vi "UHR-Fleezers Control (host) - 11.9b.vi"() -> ()   [LabVIEW 2014] (continued)
        n1088 = xnode "Read/Write Control"("FPGA VI Reference In"=w1466, "error in"=w1467, "+ phase (APD 1 Gate)"=w1464) -> ("error out"=w1465:errorcluster)  [unwired: 1 out]
      }
      event "+ phase (APD 2 Gate)", "- phase (APD 2 Gate)": Value Change {
        n1089 = event-data() -> ()  [unwired: 7 out]
        n1090 = local read "Phase Adj. (APD 2 Gate)"() -> (w1472:i16)
        n1091 = Negate(x=w1472) -> (-x=w1480:i16)
        n1092 = Select(t=w1480, s="- phase (APD 2 Gate)", f=w1472) -> (s? t:f=w1479:i16)
        n1093 = Or(x="- phase (APD 2 Gate)", y="+ phase (APD 2 Gate)") -> (x .or. y?=w1475:bool)
        n1094 = xnode "Read/Write Control"("FPGA VI Reference In"=w1482, "error in"=w1481, "Phase count adjustment (APD 2 Gate)"=w1479) -> ("FPGA VI Reference Out"=w1477:T19, "error out"=w1478:errorcluster)
        n1095 = xnode "Read/Write Control"("FPGA VI Reference In"=w1477, "error in"=w1478, "+ phase (APD 2 Gate)"=w1475) -> ("error out"=w1476:errorcluster)  [unwired: 1 out]
      }
      event "Phase Adj. (APD Acq)", "+ phase (APD Acq)", "- phase (APD Acq)": Value Change {
        n1096 = event-data() -> ()  [unwired: 7 out]
        n1097 = local read "Phase Adj. (APD Acq)"() -> (w1485:i16)
        n1098 = Negate(x=w1485) -> (-x=w1491:i16)
        n1099 = Select(t=w1491, s="+ phase (APD Acq)", f=w1485) -> (s? t:f=w1490:i16)
        n1100 = Or(x="+ phase (APD Acq)", y="- phase (APD Acq)") -> (x .or. y?=w1486:bool)
        n1101 = xnode "Read/Write Control"("FPGA VI Reference In"=w1493, "error in"=w1492, "Phase Count Adjustment (APD Acq)"=w1490) -> ("FPGA VI Reference Out"=w1488:T19, "error out"=w1489:errorcluster)
        n1102 = xnode "Read/Write Control"("FPGA VI Reference In"=w1488, "error in"=w1489, "+ phase (APD Acq)"=w1486) -> ("error out"=w1487:errorcluster)  [unwired: 1 out]
      }
      event "Phase adj. (GI)", "+ phase (GI)", "- phase (GI)": Value Change {
        n1103 = event-data() -> ()  [unwired: 7 out]
        n1104 = Negate(x="Phase adj. (GI)") -> (-x=w1502:i16)
        n1105 = Select(t=w1502, s="+ phase (GI)", f="Phase adj. (GI)") -> (s? t:f=w1501:i16)
        n1106 = Or(x="+ phase (GI)", y="- phase (GI)") -> (x .or. y?=w1497:bool)
        n1107 = xnode "Read/Write Control"("FPGA VI Reference In"=w1504, "error in"=w1503, "Phase count adjustment (GI)"=w1501) -> ("FPGA VI Reference Out"=w1499:T19, "error out"=w1500:errorcluster)
        n1108 = xnode "Read/Write Control"("FPGA VI Reference In"=w1499, "error in"=w1500, "+ phase (GI)"=w1497) -> ("error out"=w1498:errorcluster)  [unwired: 1 out]
      }
      event "Phase adj. (GI) 2", "+ phase (GI) 2", "- phase (GI) 2": Value Change {
        n1109 = event-data() -> ()  [unwired: 7 out]
        n1110 = Negate(x="Phase adj. (GI) 2") -> (-x=w1513:i16)
        n1111 = Select(t=w1513, s="+ phase (GI) 2", f="Phase adj. (GI) 2") -> (s? t:f=w1512:i16)
        n1112 = Or(x="+ phase (GI) 2", y="- phase (GI) 2") -> (x .or. y?=w1508:bool)
        n1113 = xnode "Read/Write Control"("FPGA VI Reference In"=w1515, "error in"=w1514, "Phase count adjustment (GI) 2"=w1512) -> ("FPGA VI Reference Out"=w1510:T19, "error out"=w1511:errorcluster)
        n1114 = xnode "Read/Write Control"("FPGA VI Reference In"=w1510, "error in"=w1511, "+ phase (GI) 2"=w1508) -> ("error out"=w1509:errorcluster)  [unwired: 1 out]
      }
      event "Phase adj. (Green FB)", "- phase (Green FB)", "+ phase (Green FB)": Value Change {
        n1115 = event-data() -> ()  [unwired: 7 out]
        n1116 = Negate(x="Phase adj. (Green FB)") -> (-x=w1524:i16)
        n1117 = Select(t=w1524, s="+ phase (Green FB)", f="Phase adj. (Green FB)") -> (s? t:f=w1523:i16)
        n1118 = Or(x="+ phase (Green FB)", y="- phase (Green FB)") -> (x .or. y?=w1519:bool)
        n1119 = xnode "Read/Write Control"("FPGA VI Reference In"=w1526, "error in"=w1525, "Phase count adjustment (Green FB)"=w1523) -> ("FPGA VI Reference Out"=w1521:T19, "error out"=w1522:errorcluster)
        n1120 = xnode "Read/Write Control"("FPGA VI Reference In"=w1521, "error in"=w1522, "+ phase (Green FB)"=w1519) -> ("error out"=w1520:errorcluster)  [unwired: 1 out]
      }
      event "Invert APD Gate", "APD Gate ON Count", "APD Gate OFF Count", "APD Gate", "APD Integration Time (s)", "APD 1 AO Mult.", "APD 2 AO Mult.", "On one out of X cycles": Value Change {
        n1121 = event-data() -> ()  [unwired: 7 out]
        n1122 = Add(x="GI Frequency, ON count", y="GI Frequency, OFF count") -> (x+y=w1530:u32)
        n1123 = Add(x="APD Gate ON Count", y="APD Gate OFF Count") -> (x+y=w1543:u32)
        n1124 = Multiply(x="On one out of X cycles", y=w1530) -> (x*y=w1527:u32)
        "Green FB Count" <- w1527
        n1125 = Subtract(x=w1527, y="GI Frequency, ON count") -> (x-y=w1528:u32)
        n1126 = Multiply(x=w1543, y="On one out of X cycles") -> (x*y=w1542:u32)
        n1127 = Subtract(x=w1542, y="APD Gate ON Count") -> (x-y=w1541:u32)
        n1128 = local read "DMA Update Period (s)"() -> (w1544:dbl)
        n1129 = Multiply(x="APD Integration Time (s)", y=40000000.0) -> (x*y=w1549:dbl)
        n1130 = Reciprocal(x="APD Integration Time (s)") -> (1/x=→"APD Acq Rate (Hz)":dbl)
        n1131 = To Unsigned Long Integer(number=w1549) -> (unsigned 32bit integer=w1533:u32)
        "APD Int. Count" <- w1533
        n1132 = xnode "Read/Write Control"("FPGA VI Reference In"=w1553, "error in"=w1552, "Invert APD Gate"="Invert APD Gate", "APD Gate ON Count"="APD Gate ON Count", "APD Gate OFF Count"=w1541, "APD Acq Rate Count"=w1533, "APD Gate Operating Mode"="APD Gate", "APD 1 AO scale factor"="APD 1 AO Mult.", "APD 2 AO scale factor"="APD 2 AO Mult.", "Green interlace ON count"="GI Frequency, ON count", "Green interlace OFF count"=w1528, "Green interlace ON count 2"="GI Frequency, ON count", "Green interlace OFF count 2"=w1528, "Green FB Count"=w1527) -> ("error out"=w1551:errorcluster)  [unwired: 1 out]
        n1133 = Divide(x=w1544, y="APD Integration Time (s)") -> (x/y=w1547:dbl)
        n1134 = Multiply(x=2.0, y=w1547) -> (x*y=w1546:dbl)
        n1135 = local write "APD Samples/FIFO Acq."(w1547) -> ()
        n1136 = local write "APD Elements/DMA read"(w1546) -> ()
      }
      event "Number of F/B Scans (AOD)", "Scan Speed (nm/s)", "Scan BD", "Initial D (MHz)", "Step Size (nm)", "Scan Range (nm)", "Wiggle amp 1 (units?)": Value Change {
        w1615 = 123.0  # AOM cal (nm/MHz)
        n1137 = event-data() -> ()  [unwired: 7 out]
        n1138 = local read "BD 1 Frequency 1 (MHz)"() -> (w1598:dbl)
        n1139 = local read "AOM X Cal (nm/MHz)"() -> (w1590:dbl)
        n1140 = local read "BD 2 Frequency 1 (MHz)"() -> (w1604:dbl)
        n1141 = local read "X RF Frequency Limits (MHz)"() -> (w1602:T16)
        n1142 = local read "Y RF Frequency Limits (MHz)"() -> (w1599:T16)
        n1143 = Negate(x="Scan Range (nm)") -> (-x=w1568:dbl)
        n1144 = Divide(x=w1568, y=w1590) -> (x/y=w1572:dbl)
        n1145 = Select(t=w1602, s="Scan BD", f=w1599) -> (s? t:f=w1601:T16)
        n1146 = Select(t=w1598, s="Scan BD", f=w1604) -> (s? t:f=w1603:dbl)
        n1147 = Unbundle By Name(w1601) -> ("Maximum"=w1610:dbl, "Minimum"=w1609:dbl)
        n1148 = Add(x=w1572, y=w1603) -> (x+y=w1607:dbl)
        n1149 = Divide(x=w1568, y="Step Size (nm)") -> (x/y=w1587:dbl)
        n1150 = Divide(x="Step Size (nm)", y=w1590) -> (x/y=w1596:dbl)
        n1151 = Absolute Value(x=w1587) -> (abs(x)=w1571:dbl)
        n1152 = Sign(1:w1568) -> (0:w1569:dbl)
        n1153 = In Range and Coerce(upper limit=w1610, x=w1607, lower limit=w1609) -> (coerced(x)=w1606:dbl, In Range?=w1608:bool)
        n1154 = To Unsigned Quad Integer(1:w1571) -> (0:w1586:u64)
        "Scan steps (AOD)" <- w1586
        n1155 = call "IR AOM freq to word.vi"("Frequency In (MHz)"=w1596) -> ("Frequency Word Out (double)"=w1593:dbl)
        n1156 = Multiply(x=w1569, y=w1593) -> (x*y=w1570:dbl)
        n1157 = Subtract(x=w1607, y=w1606) -> (x-y=w1605:dbl)
        n1158 = To Quad Integer(1:w1570) -> (0:w1592:i64)
        "Incr. int (AOD)" <- w1592
        n1159 = Subtract(x=w1572, y=w1605) -> (x-y=w1591:dbl)
        "Scan Range (MHz)" <- w1591
        n1160 = Select(t=w1572, s=w1608, f=w1591) -> (s? t:f=w1611:dbl)
        n1161 = Multiply(x=w1591, y=w1590) -> (x*y=w1589:dbl)
        n1162 = Decrement(x=w1586) -> (x-1=w1639:u64)
        n1163 = Negate(x=w1589) -> (-x=w1585:dbl)
        n1164 = local write "Scan Range (nm)"(w1585) -> ()
        n1165 = Divide(x=w1611, y=w1639) -> (x/y=w1595:dbl)
        "Scan Increment (MHz)" <- w1595
        n1166 = call "IR AOM freq to word.vi"("Frequency In (MHz)"=w1595) -> ("Frequency Word Out (double)"=w1594:dbl)
        n1167 = Divide(x="Step Size (nm)", y="Scan Speed (nm/s)") -> (x/y=w1582:dbl)
        n1168 = To Quad Integer(1:w1594) -> ()  [unwired: 1 out]
        n1169 = local read "Number Interlace Sets"() -> (w1566:u8)
        n1170 = local read "AI Count (ticks)"() -> (w1567:u32)
        n1171 = local read "Total Counts (ticks)"() -> (w1565:u32)
        n1172 = local read "# Samples/trap"() -> (w1597:u32)
        n1173 = Multiply(x=w1567, y=w1566) -> (x*y=w1564:u32)
        n1174 = Divide(x=w1565, y=w1564) -> (x/y=w1563:dbl)
        n1175 = Select(t=w1598, s="Scan BD", f=w1604) -> (s? t:f=w1636:dbl)
        "Initial freq. (MHz)" <- w1636
        n1176 = Add(x=w1611, y=w1636) -> (x+y=→"Final freq. (MHz)":dbl)
        n1177 = Divide(x=w1565, y=40000000.0) -> (x/y=w1581:dbl)
        n1178 = Divide(x=w1582, y=w1581) -> (x/y=w1580:dbl)
        n1179 = To Unsigned Quad Integer(1:w1580) -> (0:w1555:u64)
        n1180 = Quotient & Remainder(x=w1555, y=u64 2) -> (x-y*floor(x/y)=w1559:u64)  [unwired: 1 out]
        n1181 = Equal?(x=w1559, y=u64 0) -> (x = y?=w1557:bool)
        n1182 = Decrement(x=w1555) -> (x-1=w1556:u64)
        n1183 = Select(t=w1555, s=w1557, f=w1556) -> (s? t:f=w1554:u64)
        "Cycles/step (AOD)" <- w1554
        n1184 = xnode "Read/Write Control"("FPGA VI Reference In"=w1647, "error in"=w1646, "Scan steps"=w1586, "Number of scans"="Number of F/B Scans (AOD)", "Cycles per step"=w1554, "Scan freq.  increment"=w1592, "Scan BD"="Scan BD") -> ("error out"=w1645:errorcluster)  [unwired: 1 out]
        n1185 = Multiply(x=w1586, y=w1554) -> (x*y=w1640:u64)
        n1186 = Multiply(x=w1640, y=u64 2) -> (x*y=w1562:u64)
        n1187 = Multiply(x=w1563, y=w1562) -> (x*y=w1561:dbl)
        "Data points/scan (f/b)" <- w1561
        n1188 = Multiply(x=w1561, y="Number of F/B Scans (AOD)") -> (x*y=w1643:dbl)
        "Data points/scans" <- w1643
        n1189 = Divide(x=w1643, y=w1597) -> (x/y=→"N sets should be saved":dbl)
        n1190 = Multiply(x=w1640, y=w1581) -> (x*y=w1579:dbl)
        "Time/Scan (s) (AOD)" <- w1579
        n1191 = Select(t=w1611, s="Scan BD", f=0.0) -> (s? t:f=w1637:dbl)
        n1192 = Select(t=0.0, s="Scan BD", f=w1611) -> (s? t:f=w1633:dbl)
        n1193 = local read "BD 2 Frequency 2 (MHz)"() -> (w1629:dbl)
        n1194 = local read "BD 1 Frequency 2 (MHz)"() -> (w1632:dbl)
        n1195 = Add(x=w1633, y=w1604) -> (x+y=w1630:dbl)
        n1196 = Add(x=w1598, y=w1637) -> (x+y=w1631:dbl)
        n1197 = Multiply(x=w1579, y=2.0) -> (x*y=w1578:dbl)
        n1198 = Multiply(x=w1578, y="Number of F/B Scans (AOD)") -> (x*y=w1575:dbl)
        n1199 = Divide(x=w1575, y=60.0) -> (x/y=→"Time to Finish All (min)":dbl)
        n1200 = Add(x="Trap 2 Bead Size (nm)", y="Trap 1 Bead Size (nm)") -> (x+y=w1619:dbl)
        n1201 = Divide(x=w1619, y=2.0) -> (x/y=w1613:dbl)
        n1202 = Subtract(x=w1630, y=w1629) -> (x-y=w1627:dbl)
        n1203 = Subtract(x=w1631, y=w1632) -> (x-y=w1628:dbl)
        n1204 = local read "Initial D (MHz)"() -> (w1616:dbl)
        n1205 = Square(x=w1627) -> (x^2=w1626:dbl)
        n1206 = Square(x=w1628) -> (x^2=w1625:dbl)
        n1207 = Add(x=w1625, y=w1626) -> (x+y=w1624:dbl)
        n1208 = Square Root(x=w1624) -> (sqrt(x)=w1623:dbl)
        "Final D (MHz)" <- w1623
        n1209 = Multiply(x=w1615, y=w1623) -> (x*y=w1622:dbl)
        n1210 = Multiply(x=w1616, y=w1615) -> (x*y=w1614:dbl)
        n1211 = Subtract(x=w1614, y=w1613) -> (x-y=→"Initial sep (nm)":dbl)
        n1212 = Subtract(x=w1622, y=w1613) -> (x-y=→"Final sep (nm)":dbl)
      }
      event "Freq or Amp switch first", "Swap F1 and F2", "Freq switch delay", "Amp switch delay": Value Change {
        n1213 = event-data() -> ()  [unwired: 7 out]
        n1214 = local read "Freq or Amp switch first"() -> (w1648:bool)
        n1215 = local read "Amp switch delay"() -> (w1649:u16)
        n1216 = local read "Freq switch delay"() -> (w1651:u16)
        n1217 = local read "Swap F1 and F2"() -> (w1650:bool)
        n1218 = xnode "Read/Write Control"("FPGA VI Reference In"=w1654, "error in"=w1653, "Freq switch delay"=w1651, "Swap F1 and F2"=w1650, "Amp switch delay"=w1649, "Freq or Amp switch first"=w1648) -> ("error out"=w1652:errorcluster)  [unwired: 1 out]
      }
      event "Scan steps (MCL)", "Number of scans (MCL)", "Scan Range (V)\n(of steps)", "2D or 1D Scan", "N APD Samp/step", "Fast Scan Dir", "Continuous MCL Scanning", "Scan lines (y)": Value Change {
        w1656 = 32767.0 ("y")
        n1219 = event-data() -> ()  [unwired: 7 out]
        n1220 = Select(t="Scan lines (y)", s="2D or 1D Scan", f="Number of scans (MCL)") -> (s? t:f=w1661:u64)
        n1221 = Decrement(x="Scan steps (MCL)") -> (x-1=w1677:u64)
        n1222 = Divide(x="Scan Range (V)\n(of steps)", y=w1677) -> (x/y=w1676:dbl)
        "Desired Scan Incr (V)" <- w1676
        n1223 = local read "APD Integration Time (s)"() -> (w1669:dbl)
        n1224 = Multiply(x=w1676, y=w1656) -> (x*y=w1685:dbl)
        n1225 = Divide(x=w1685, y=10.0) -> (x/y=w1675:dbl)
        "Desired incr (int)" <- w1675
        n1226 = local read "Update Count (MCL)"() -> (w1681:u32)
        n1227 = Round Toward -Infinity(1:w1675) -> (0:w1684:dbl)
        n1228 = To Word Integer(number=w1684) -> (16bit integer=w1659:i16)
        "Actual Incr. int (MCL)" <- w1659
        n1229 = Multiply(x=w1669, y=40000000.0) -> (x*y=w1682:dbl)
        n1230 = Divide(x=w1682, y=w1681) -> (x/y=w1680:dbl)
        n1231 = Multiply(x=i16 10, y=w1659) -> (x*y=w1657:i16)
        n1232 = Multiply(x="N APD Samp/step", y=w1680) -> (x*y=w1679:dbl)
        "Cycles/step (MCL)" <- w1679
        n1233 = Divide(x=w1657, y=w1656) -> (x/y=→"Actual MCL Inc (V)":dbl)
        n1234 = Multiply(x="N APD Samp/step", y="Scan steps (MCL)") -> (x*y=w1671:dbl)
        n1235 = local read "APD Samples/FIFO Acq."() -> (w1668:dbl)
        n1236 = Multiply(x=w1671, y=u64 2) -> (x*y=w1670:dbl)
        "Data points/scan (f+b)" <- w1670
        n1237 = Multiply(x=w1670, y=w1661) -> (x*y=w1688:dbl)
        "Data points/scans (MCL)" <- w1688
        n1238 = Multiply(x=w1669, y=w1670) -> (x*y=w1662:dbl)
        "Time/f+b scan (s) (MCL)" <- w1662
        n1239 = Divide(x=w1688, y=w1668) -> (x/y=→"N sets should be saved (MCL)":dbl)
        n1240 = Multiply(x=w1662, y=w1661) -> (x*y=→"Total Time (s)":dbl)
        n1241 = Not(x="Fast Scan Dir") -> (.not. x?=w1666:bool)
        n1242 = xnode "Read/Write Control"("FPGA VI Reference In"=w1692, "error in"=w1691, "Scan steps (MCL)"="Scan steps (MCL)", "Number of scans (MCL)"=w1661, "Cycles per step (MCL)"=w1679, "Scan freq.  increment (MCL)"=w1659, "1D or 2D Scan?"="2D or 1D Scan", "MCL Scan Axis"=w1666, "Cont. Scan (MCL)"="Continuous MCL Scanning") -> ("error out"=w1690:errorcluster)  [unwired: 1 out]
      }
      event "Read Cal": Value Change {
        w1694 = 1000.0 ("y")
        n1243 = event-data() -> ()  [unwired: 7 out]
        n1244 = local read "Save file name"() -> (w1719:path)
        n1245 = local write "Read Cal"(FALSE ("Read Cal")) -> ()
        n1246 = Strip Path(path=w1719) -> (stripped path=w1718:path)  [unwired: 1 out]
        n1247 = Path To String(path=w1718) -> (string=w1717:string)
        n1248 = Concatenate Strings(w1717, "\\current.cal" ("string")) -> (w1715:string)
        n1249 = String To Path(string=w1715) -> (path=w1714:path)
        n1250 = Open/Create/Replace File(file path (use dialog)=w1714, operation (0:open)=T25."open", access (0:read/write)=enum16{"read/write", "read-only", "write-only"}."read-only") -> (refnum out=w1722:refnum<file>, error out=w1708:errorcluster)  [unwired: 1 in, 3 out]
        n1251 = Deny Access(4:w1708, 7:w1722) -> (0:w1707:errorcluster, 3:w1713:refnum<file>)  [unwired: 1 out]
        n1252 = Read from Binary File(5:0.0, 8:w1707, 9:T24."big-endian, network order" ("byte order (0:big-endian, network order)"), 10:-1 ("count (1)"), 11:w1713) -> (0:w1706:errorcluster, 2:w1704:dbl[], 3:w1709:refnum<file>)  [unwired: 2 out]
        n1253 = Array To Cluster(array=w1704) -> (cluster=w1703:T27)
        n1254 = Unbundle(w1703) -> ("[0]"=w1702:dbl, "[1]"=w1701:dbl, "[2]"=w1700:dbl, "[3]"=w1699:dbl, "[4]"=w1698:dbl, "[5]"=w1697:dbl)
        n1255 = Close File(refnum=w1709, error in=w1706) -> (error out=→"Read cal error":errorcluster)  [unwired: 1 out]
        n1256 = Multiply(x=w1697, y=w1694) -> (x*y=w1695:dbl)
        n1257 = local write "T2 k_x (pN/nm)"(w1699) -> ()
        n1258 = local write "T1 k_x (pN/nm)"(w1700) -> ()
        n1259 = local write "T1 a_x (nm/V)"(w1702) -> ()
        n1260 = local write "T2 a_x (nm/V)"(w1701) -> ()
        n1261 = Multiply(x=w1698, y=w1694) -> (x*y=w1696:dbl)
        n1262 = local write "T1 offset_x (mV)"(w1696) -> ()
        n1263 = local write "T2 offset_x (mV)"(w1695) -> ()
      }
      event "Read FX file": Value Change {
        n1264 = event-data() -> ()  [unwired: 7 out]
        n1265 = local write "Read FX file"(FALSE ("Read residual")) -> ()
        n1266 = local read "Save file name"() -> (w1747:path)
        n1267 = Strip Path(path=w1747) -> (stripped path=w1746:path)  [unwired: 1 out]
        n1268 = Path To String(path=w1746) -> (string=w1745:string)
        n1269 = Concatenate Strings(w1745, "\\current.cal" ("string")) -> (w1743:string)
        n1270 = String To Path(string=w1743) -> (path=w1742:path)
        n1271 = Open/Create/Replace File(file path (use dialog)=w1742, operation (0:open)=T25."open", access (0:read/write)=enum16{"read/write", "read-only", "write-only"}."read-only") -> (refnum out=w1739:refnum<file>, error out=w1736:errorcluster)  [unwired: 3 in, 1 out]
        n1272 = Deny Access(4:w1736, 7:w1739) -> (0:w1735:errorcluster, 3:w1738:refnum<file>)  [unwired: 1 in]
        n1273 = Read from Binary File(5:0.0, 8:w1735, 9:T24."big-endian, network order" ("byte order (0:big-endian, network order)"), 10:-1 ("count"), 11:w1738) -> (0:w1731:errorcluster, 2:w1725:dbl[], 3:w1732:refnum<file>)  [unwired: 1 in, 1 out]
        n1274 = Index Array(array=w1725, index=6) -> (element=→"Bad fit error":dbl)
        n1275 = Index Array(array=w1725, index=7) -> (element=→"Fit offset":dbl)
        n1276 = Index Array(array=w1725, index=8) -> (element=→"Hyst. error":dbl)
        n1277 = Close File(refnum=w1732, error in=w1731) -> ()  [unwired: 2 out]
      }
      event "Abort MCL Scan": Value Change {
        n1278 = event-data() -> ()  [unwired: 7 out]
        n1279 = local write "MCL Scanning"(FALSE ("MCL Scanning")) -> ()
        n1280 = xnode "Read/Write Control"("FPGA VI Reference In"=w1752, "error in"=w1751, "Abort scan (MCL)"="Abort MCL Scan") -> ("error out"=w1750:errorcluster)  [unwired: 1 out]
      }
      event "Update Count (MCL)": Value Change {
        n1281 = event-data() -> ()  [unwired: 7 out]
        n1282 = xnode "Read/Write Control"("FPGA VI Reference In"=w1756, "error in"=w1755, "MCL count"="Update Count (MCL)") -> ("error out"=w1754:errorcluster)  [unwired: 1 out]
      }
      event "Phase adjust (MCL)", "+ phase (MCL)", "- phase (MCL)": Value Change {
        n1283 = event-data() -> ()  [unwired: 7 out]
        n1284 = Negate(x="Phase adjust (MCL)") -> (-x=w1765:i16)
        n1285 = Select(t=w1765, s="- phase (MCL)", f="Phase adjust (MCL)") -> (s? t:f=w1763:i16)
        n1286 = Or(x="- phase (MCL)", y="+ phase (MCL)") -> (x .or. y?=w1758:bool)
        n1287 = xnode "Read/Write Control"("FPGA VI Reference In"=w1767, "error in"=w1766, "Phase count adjustment (MCL)"=w1763) -> ("FPGA VI Reference Out"=w1759:T19, "error out"=w1760:errorcluster)
        n1288 = xnode "Read/Write Control"("FPGA VI Reference In"=w1759, "error in"=w1760, "+ phase (MCL)"=w1758) -> ("error out"=w1757:errorcluster)  [unwired: 1 out]
      }
      event "Abort AOD Scan": Value Change {
        n1289 = event-data() -> ()  [unwired: 7 out]
        n1290 = xnode "Read/Write Control"("FPGA VI Reference In"=w1771, "error in"=w1770, "Abort scan"="Abort AOD Scan") -> ("error out"=w1769:errorcluster)  [unwired: 1 out]
      }
      event "Continuous AOD Scanning": Value Change {
        n1291 = event-data() -> ()  [unwired: 7 out]
        n1292 = xnode "Read/Write Control"("FPGA VI Reference In"=w1775, "error in"=w1774, "Cont. Scan"="Continuous AOD Scanning") -> ("error out"=w1773:errorcluster)  [unwired: 1 out]
      }
      event "Index": Value Change {
        n1293 = event-data() -> ()  [unwired: 7 out]
        n1294 = call "Create new save file.vi"("Insert"="", "Ext"=".dat" ("string"), "Index In"="Index") -> ("Path Out"=→"Save file name":path, "Index Out"=w1776:dbl)
        "Save index" <- w1776
        n1295 = local write "Index"(w1776) -> ()
      }
      event "AO1", "AO2": Value Change {
        w1791 = 10.0 ("y")
        w1790 = 32767.0 ("y")
        n1296 = event-data() -> ()  [unwired: 7 out]
        n1297 = local read "AO2"() -> (w1789:dbl)
        n1298 = local read "AO1"() -> (w1786:dbl)
        n1299 = Multiply(x=w1786, y=w1790) -> (x*y=w1785:dbl)
        n1300 = Multiply(x=w1789, y=w1790) -> (x*y=w1788:dbl)
        n1301 = Divide(x=w1785, y=w1791) -> (x/y=w1784:dbl)
        n1302 = Divide(x=w1788, y=w1791) -> (x/y=w1787:dbl)
        n1303 = To Word Integer(number=w1784) -> (16bit integer=w1792:i16)
        n1304 = To Word Integer(number=w1787) -> (16bit integer=w1793:i16)
        n1305 = xnode "Read/Write Control"("FPGA VI Reference In"=w1783, "error in"=w1782, "AO1"=w1792, "AO2"=w1793) -> ("error out"=w1781:errorcluster)  [unwired: 1 out]
      }
      event "Inject Pump 1": Value Change {
        n1306 = event-data() -> ()  [unwired: 7 out]
        n1307 = local read "Use Harvard pumps\nfor beads (else Chemyx)"() -> (w1795:bool)
        n1308 = case shown="True" w1795 {
          tunnel: "Inject Pump 1" -> [w1799 w1837]
          tunnel: w1794 -> [_ w1838]
          frame False {
            n1309 = local read "Pump write delay (ms)"() -> (w1798:dbl)
            n1310 = local read "Chemyx Syringe Pump Serial Port"() -> (w1797:refnum<visa-resource-name>)
            n1311 = case shown="True" w1799 {
              tunnel: w1798 -> [w1805 w1819]
              tunnel: w1797 -> [w1802 w1818]
              frame False {
                n1312 = flat-sequence {
                  tunnel: w1802 -> [w1806]
                  tunnel: [w1806] -> w1803
                  tunnel: w1805 -> [_]
                  tunnel: [w1809] -> w1804
                  tunnel: w1803 -> [w1809]
                  tunnel: w1804 -> [w1810]
                  tunnel: [w1810] -> w1800
                  tunnel: [w1812] -> w1801
                  tunnel: w1800 -> [w1812]
                  tunnel: w1801 -> [w1814]
                  frame #0 {
                    n1313 = call "Write to pump.vi"("string"="enter pump1", "VISA resource name"=w1806) -> ()  [unwired: 1 out]
                  }
                  frame #1 {
                    n1314 = Wait (ms)(milliseconds to wait="Pump pause delay (ms)") -> ()  [unwired: 1 out]
                  }
                  frame #2 {
                    n1315 = call "Write to pump.vi"("string"="stop", "VISA resource name"=w1810) -> ()  [unwired: 1 out]
                  }
                  frame #3 {
                    n1316 = Wait (ms)(milliseconds to wait=u32 500) -> ()  [unwired: 1 out]
                  }
                  frame #4 {
                    n1317 = call "Write to pump.vi"("string"="stop", "VISA resource name"=w1814) -> ()  [unwired: 1 out]
                  }
                }
              }
              frame True {
                n1318 = flat-sequence {
                  tunnel: w1818 -> [w1828]
                  tunnel: w1819 -> [w1823]
                  tunnel: w1819 -> [w1830]
                  tunnel: w1818 -> [w1831]
                  tunnel: [w1831] -> w1816
                  tunnel: [w1833] -> w1817
                  tunnel: w1816 -> [w1833]
                  tunnel: w1817 -> [w1835]
                  frame #0 {
                    n1319 = local read "All Pump Parameters"() -> (w1822:T5)
                    n1320 = Unbundle By Name(w1822) -> ("Pump 1"=w1829:T28)
                    n1321 = call "Set pump parameters.vi"("Pump write delay (ms)"=w1823, "Volume (uL)"="Ch 1 Inject Volume (uL)", "Rate (uL/h)"="Ch 1 Inject Rate (ul/h)", "Units"=4.0, "Pump #"=1.0, "Pump Parameters In"=w1829, "VISA resource name"=w1828) -> ("Pump Parameters Out"=w1821:T28)  [unwired: 3 in]
                    n1322 = Bundle By Name(cluster=w1822, "Pump 1"=w1821) -> (w1820:T5)
                    n1323 = local write "All Pump Parameters"(w1820) -> ()
                  }
                  frame #1 {
                    n1324 = Wait (ms)(milliseconds to wait=w1830) -> ()  [unwired: 1 out]
                  }
                  frame #2 {
                    n1325 = call "Write to pump.vi"("string"="start", "VISA resource name"=w1831) -> ()  [unwired: 1 out]
                  }
                  frame #3 {
                    n1326 = Wait (ms)(milliseconds to wait=u32 500) -> ()  [unwired: 1 out]
                  }
                  frame #4 {
                    n1327 = call "Write to pump.vi"("string"="start", "VISA resource name"=w1835) -> ()  [unwired: 1 out]
                  }
                }
              }
            }
          }
          frame True {
            n1328 = case shown="True" w1837 {
              tunnel: w1838 -> [w1839 w1849]
              frame False {
                n1329 = flat-sequence {
                  tunnel: w1839 -> [w1841]
                  frame #0 {
                    n1330 = local write "Flushing P1"(FALSE ("Flushing P1")) -> ()
                    n1331 = Concatenate Strings("stop" ("string"), "\r") -> (w1843:string)
                    n1332 = VISA Write(VISA resource name=w1841, write buffer=w1843) -> ()  [unwired: 1 in, 3 out]
                  }
                  frame #1 {
                    n1333 = property on="Clear Volume P1" class="Bool (strict)"("Val(Sgnl)"=TRUE ("Value (Signaling)")) -> ()  [unwired: 2 in, 2 out]
                  }
                }
              }
              frame True {
                n1334 = local read "Normal Flow Rate (ul/h) P1"() -> (w1847:dbl)
                n1335 = Number To Decimal String(number=w1847) -> (decimal integer string=w1853:string)  [unwired: 1 in]
                n1336 = Concatenate Strings("irate  " ("string"), w1853, " u/h" ("string"), "\r") -> (w1851:string)
                n1337 = VISA Write(VISA resource name=w1849, write buffer=w1851) -> (VISA resource name out=w1848:refnum<visa-resource-name>)  [unwired: 1 in, 2 out]
                n1338 = Concatenate Strings("irun" ("string"), "\r") -> (w1855:string)
                n1339 = VISA Write(VISA resource name=w1848, write buffer=w1855) -> ()  [unwired: 1 in, 3 out]
              }
            }
          }
        }
      }
      event "Inject Pump 3": Value Change {
        n1340 = event-data() -> ()  [unwired: 7 out]
        n1341 = local read "Use Harvard pumps\nfor beads (else Chemyx)"() -> (w1858:bool)
        n1342 = case shown="True" w1858 {
          tunnel: "Inject Pump 3" -> [w1862 w1901]
          tunnel: w1857 -> [_ w1900]
          frame False {
            n1343 = local read "Pump write delay (ms)"() -> (w1861:dbl)
            n1344 = case shown="True" w1862 {
              tunnel: w1861 -> [w1868 w1882]
              tunnel: "Chemyx Syringe Pump Serial Port" -> [w1865 w1881]
              frame False {
                n1345 = flat-sequence {
                  tunnel: w1865 -> [w1869]
                  tunnel: [w1869] -> w1866
                  tunnel: w1868 -> [_]
                  tunnel: [w1872] -> w1867
                  tunnel: w1866 -> [w1872]
                  tunnel: w1867 -> [w1873]
                  tunnel: [w1873] -> w1863
                  tunnel: [w1875] -> w1864
                  tunnel: w1863 -> [w1875]
                  tunnel: w1864 -> [w1877]
                  frame #0 {
                    n1346 = call "Write to pump.vi"("string"="enter pump3", "VISA resource name"=w1869) -> ()  [unwired: 1 out]
                  }
                  frame #1 {
                    n1347 = local read "Pump pause delay (ms)"() -> (w1871:u32)
                    n1348 = Wait (ms)(milliseconds to wait=w1871) -> ()  [unwired: 1 out]
                  }
                  frame #2 {
                    n1349 = call "Write to pump.vi"("string"="stop", "VISA resource name"=w1873) -> ()  [unwired: 1 out]
                  }
                  frame #3 {
                    n1350 = Wait (ms)(milliseconds to wait=u32 0) -> ()  [unwired: 1 out]
                  }
                  frame #4 {
                    n1351 = call "Write to pump.vi"("string"="stop", "VISA resource name"=w1877) -> ()  [unwired: 1 out]
                  }
                }
              }
              frame True {
                n1352 = flat-sequence {
                  tunnel: w1881 -> [w1891]
                  tunnel: w1882 -> [w1886]
                  tunnel: w1882 -> [w1893]
                  tunnel: w1881 -> [w1894]
                  tunnel: [w1894] -> w1880
                  tunnel: [w1897] -> w1879
                  tunnel: w1880 -> [w1897]
                  tunnel: w1879 -> [w1898]
                  frame #0 {
                    n1353 = local read "All Pump Parameters"() -> (w1885:T5)
                    n1354 = Unbundle By Name(w1885) -> ("Pump 3"=w1892:T28)
                    n1355 = call "Set pump parameters.vi"("Pump write delay (ms)"=w1886, "Volume (uL)"="Ch 3 Inject Volume (uL)", "Rate (uL/h)"="Ch 3 Inject Rate (ul/h)", "Units"=4.0, "Pump #"=3.0, "Pump Parameters In"=w1892, "VISA resource name"=w1891) -> ("Pump Parameters Out"=w1884:T28)  [unwired: 3 in]
                    n1356 = Bundle By Name(cluster=w1885, "Pump 3"=w1884) -> (w1883:T5)
                    n1357 = local write "All Pump Parameters"(w1883) -> ()
                  }
                  frame #1 {
                    n1358 = Wait (ms)(milliseconds to wait=w1893) -> ()  [unwired: 1 out]
                  }
                  frame #2 {
                    n1359 = call "Write to pump.vi"("string"="start", "VISA resource name"=w1894) -> ()  [unwired: 1 out]
                  }
                  frame #3 {
                    n1360 = Wait (ms)(milliseconds to wait=u32 500) -> ()  [unwired: 1 out]
                  }
                  frame #4 {
                    n1361 = call "Write to pump.vi"("string"="start", "VISA resource name"=w1898) -> ()  [unwired: 1 out]
                  }
                }
              }
            }
          }
          frame True {
            n1362 = case shown="True" w1901 {
              tunnel: w1900 -> [w1902 w1909]
              frame False {
                n1363 = flat-sequence {
                  tunnel: w1902 -> [w1904]
                  frame #0 {
                    n1364 = local write "Flushing P3"(FALSE ("Flushing P3")) -> ()
                    n1365 = Concatenate Strings("stop" ("string"), "\r") -> (w1906:string)
                    n1366 = VISA Write(VISA resource name=w1904, write buffer=w1906) -> ()  [unwired: 1 in, 3 out]
                  }
                  frame #1 {
                    n1367 = property on="Clear Volume P3" class="Bool (strict)"("Val(Sgnl)"=TRUE ("Value (Signaling)")) -> ()  [unwired: 2 in, 2 out]
                  }
                }
              }
              frame True {
                n1368 = local read "Normal Flow Rate (ul/h) P3"() -> (w1910:dbl)
                n1369 = Number To Decimal String(number=w1910) -> (decimal integer string=w1916:string)  [unwired: 1 in]
                n1370 = Concatenate Strings("irate  " ("string"), w1916, " u/h" ("string"), "\r") -> (w1914:string)
                n1371 = VISA Write(VISA resource name=w1909, write buffer=w1914) -> (VISA resource name out=w1912:refnum<visa-resource-name>)  [unwired: 1 in, 2 out]
                n1372 = Concatenate Strings("irun" ("string"), "\r") -> (w1918:string)
                n1373 = VISA Write(VISA resource name=w1912, write buffer=w1918) -> ()  [unwired: 1 in, 3 out]
              }
            }
          }
        }
      }
      event "Inject Pump 2": Value Change {
        n1374 = event-data() -> ()  [unwired: 7 out]
        n1375 = local read "Pump write delay (ms)"() -> (w1922:dbl)
        n1376 = local read "Chemyx Syringe Pump Serial Port"() -> (w1920:refnum<visa-resource-name>)
        n1377 = flat-sequence {
          tunnel: w1920 -> [w1935]
          tunnel: w1922 -> [w1931]
          tunnel: "Inject Pump 2" -> [_]
          tunnel: w1922 -> [w1937]
          tunnel: w1920 -> [w1938]
          frame #0 {
            n1378 = local read "All Pump Parameters"() -> (w1930:T5)
            n1379 = Multiply(x=60.0, y="Flush Center Ch Rate (ul/m)") -> (x*y=w1927:dbl)
            n1380 = Unbundle By Name(w1930) -> ("Pump 2"=w1936:T28)
            n1381 = call "Set pump parameters.vi"("Pump write delay (ms)"=w1931, "Volume (uL)"="Flush Center Ch Volume (uL)", "Rate (uL/h)"=w1927, "Units"=3.0, "Pump #"=2.0, "Pump Parameters In"=w1936, "VISA resource name"=w1935) -> ("Pump Parameters Out"=w1929:T28)  [unwired: 3 in]
            n1382 = Bundle By Name(cluster=w1930, "Pump 2"=w1929) -> (w1928:T5)
            n1383 = Add(x="Flush Center Ch Volume (uL)", y="Total Volume\nFlushed (uL)") -> (x+y=w1924:dbl)
            n1384 = local write "All Pump Parameters"(w1928) -> ()
            n1385 = local write "Total Volume\nFlushed (uL)"(w1924) -> ()
          }
          frame #1 {
            n1386 = Wait (ms)(milliseconds to wait=w1937) -> ()  [unwired: 1 out]
          }
          frame #2 {
            n1387 = call "Write to pump.vi"("string"="start", "VISA resource name"=w1938) -> ()  [unwired: 1 out]
          }
        }
      }
      event "Sample Channel\nFlow": Value Change {
        n1388 = event-data() -> ()  [unwired: 7 out]
        n1389 = case shown="True" "Sample Channel\nFlow" {
          tunnel: w1941 -> [w1942 w1948]
          frame False {
            n1390 = flat-sequence {
              tunnel: w1942 -> [w1944]
              frame #0 {
                n1391 = local write "Flushing samp"(FALSE ("Flushing samp")) -> ()
                n1392 = Concatenate Strings("stop" ("string"), "\r") -> (w1947:string)
                n1393 = VISA Write(VISA resource name=w1944, write buffer=w1947) -> ()  [unwired: 1 in, 3 out]
              }
            }
          }
          frame True {
            n1394 = local read "Normal Flow rate (mL/h)"() -> (w1958:dbl)
            n1395 = Number To Decimal String(number=w1958) -> (decimal integer string=w1957:string)  [unwired: 1 in]
            n1396 = Concatenate Strings("irate " ("string"), w1957, " u/h" ("string"), "\r") -> (w1953:string)
            n1397 = VISA Write(VISA resource name=w1948, write buffer=w1953) -> (VISA resource name out=w1952:refnum<visa-resource-name>)  [unwired: 1 in, 2 out]
            n1398 = Concatenate Strings("irun" ("string"), "\r") -> (w1949:string)
            n1399 = VISA Write(VISA resource name=w1952, write buffer=w1949) -> ()  [unwired: 1 in, 3 out]
          }
        }
      }
      event "Start Flow": Value Change {
        n1400 = event-data() -> ()  [unwired: 7 out]
        n1401 = local write "Sample Channel\nFlow"(TRUE ("Sample Channel\nFlow")) -> ()
        n1402 = local write "Start Flow"(FALSE ("Start Flow")) -> ()
        n1403 = Concatenate Strings("irun" ("string"), "\r") -> (w1963:string)
        n1404 = VISA Write(VISA resource name=w1959, write buffer=w1963) -> ()  [unwired: 1 in, 3 out]
      }
      event "Stop Flow": Value Change {
        w1965 = FALSE ("Stop Flow")
        n1405 = event-data() -> ()  [unwired: 7 out]
        n1406 = local write "Stop Flow"(w1965) -> ()
        n1407 = local write "Sample Channel\nFlow"(w1965) -> ()
        n1408 = Concatenate Strings("stop" ("string"), "\r") -> (w1968:string)
        n1409 = VISA Write(VISA resource name=w1966, write buffer=w1968) -> ()  [unwired: 1 in, 3 out]
      }
      event "Normal Flow rate (mL/h)": Value Change {
        n1410 = event-data() -> ()  [unwired: 7 out]
        n1411 = Number To Decimal String(number="Normal Flow rate (mL/h)") -> (decimal integer string=w1975:string)  [unwired: 1 in]
        n1412 = Concatenate Strings("irate  " ("string"), w1975, " u/h" ("string"), "\r") -> (w1974:string)
        n1413 = VISA Write(VISA resource name=w1971, write buffer=w1974) -> ()  [unwired: 1 in, 3 out]
      }
      event "Flush Sample": Value Change {
        n1414 = event-data() -> ()  [unwired: 7 out]
        n1415 = flat-sequence {
          tunnel: w1977 -> [w2005]
          frame #0 {
            # "set parameters (rate, volume) for flush, clear volume"
            n1416 = Number To Decimal String(number="Flush rate (mL/m)") -> (decimal integer string=w2001:string)  [unwired: 1 in]
            n1417 = local write "Sample Channel\nFlow"(TRUE ("Sample Channel\nFlow")) -> ()
            n1418 = Concatenate Strings("irate  " ("string"), w2001, " u/m" ("string"), "\r") -> (w2003:string)
            n1419 = VISA Write(VISA resource name=w2005, write buffer=w2003) -> (VISA resource name out=w1999:refnum<visa-resource-name>)  [unwired: 1 in, 2 out]
            n1420 = Number To Decimal String(number="Flush volume (mL)") -> (decimal integer string=w1990:string)  [unwired: 1 in]
            n1421 = Reciprocal(x="Flush rate (mL/m)") -> (1/x=w1984:dbl)
            n1422 = Concatenate Strings("tvolume  " ("string"), w1990, " u" ("string"), "\r") -> (w1988:string)
            n1423 = Multiply(x=w1984, y="Flush volume (mL)") -> (x*y=w1982:dbl)
            n1424 = VISA Write(VISA resource name=w1999, write buffer=w1988) -> (VISA resource name out=w1987:refnum<visa-resource-name>)  [unwired: 1 in, 2 out]
            n1425 = Multiply(x=w1982, y=60.0) -> (x*y=→"Samp Flush Time (s)":dbl)
            n1426 = Concatenate Strings("cvolume" ("string"), "\r") -> (w1986:string)
            n1427 = VISA Write(VISA resource name=w1987, write buffer=w1986) -> (VISA resource name out=w1997:refnum<visa-resource-name>)  [unwired: 1 in, 2 out]
            n1428 = Concatenate Strings("irun" ("string"), "\r") -> (w1995:string)
            n1429 = VISA Write(VISA resource name=w1997, write buffer=w1995) -> ()  [unwired: 1 in, 3 out]
          }
          frame #1 {
            "Flushing samp" <- TRUE ("Boolean")
          }
        }
      }
      event "Flush Pump 3": Value Change {
        n1430 = event-data() -> ()  [unwired: 7 out]
        n1431 = flat-sequence {
          tunnel: w2007 -> [w2010]
          frame #0 {
            # "set paramaters (rate, volume) for flush, clear volume"
            n1432 = Number To Decimal String(number="Flush rate (uL/m) P3") -> (decimal integer string=w2032:string)  [unwired: 1 in]
            n1433 = local write "Inject Pump 3"(TRUE ("Inject Pump 3")) -> ()
            n1434 = Concatenate Strings("irate  " ("string"), w2032, " u/m" ("string"), "\r") -> (w2034:string)
            n1435 = VISA Write(VISA resource name=w2010, write buffer=w2034) -> (VISA resource name out=w2030:refnum<visa-resource-name>)  [unwired: 1 in, 2 out]
            n1436 = Reciprocal(x="Flush rate (uL/m) P3") -> (1/x=w2014:dbl)
            n1437 = Number To Decimal String(number="Volume (uL) P3") -> (decimal integer string=w2021:string)  [unwired: 1 in]
            n1438 = Multiply(x="Volume (uL) P3", y=w2014) -> (x*y=w2013:dbl)
            n1439 = Concatenate Strings("tvolume  " ("string"), w2021, " u" ("string"), "\r") -> (w2019:string)
            n1440 = Multiply(x=w2013, y=60.0) -> (x*y=→"HP3 Flush Time (s)":dbl)
            n1441 = VISA Write(VISA resource name=w2030, write buffer=w2019) -> (VISA resource name out=w2018:refnum<visa-resource-name>)  [unwired: 1 in, 2 out]
            n1442 = Concatenate Strings("cvolume" ("string"), "\r") -> (w2017:string)
            n1443 = VISA Write(VISA resource name=w2018, write buffer=w2017) -> (VISA resource name out=w2028:refnum<visa-resource-name>)  [unwired: 1 in, 2 out]
            n1444 = Concatenate Strings("irun" ("string"), "\r") -> (w2026:string)
            n1445 = VISA Write(VISA resource name=w2028, write buffer=w2026) -> ()  [unwired: 1 in, 3 out]
          }
          frame #1 {
            "Flushing P3" <- TRUE ("Flushing P3")
          }
        }
      }
      event "Flush Pump 1": Value Change {
        n1446 = event-data() -> ()  [unwired: 7 out]
        n1447 = flat-sequence {
          tunnel: [w2048] -> w2038
          tunnel: w2037 -> [w2041]
          tunnel: w2038 -> [_]
          frame #0 {
            # "set paramaters (rate, volume) for flush, clear volume"
            n1448 = local write "Inject Pump 1"(TRUE ("Inject Pump 1")) -> ()
            n1449 = Number To Decimal String(number="Flush rate (uL/m) P1") -> (decimal integer string=w2064:string)  [unwired: 1 in]
            n1450 = Concatenate Strings("irate  " ("string"), w2064, " u/m" ("string"), "\r") -> (w2066:string)
            n1451 = VISA Write(VISA resource name=w2041, write buffer=w2066) -> (VISA resource name out=w2062:refnum<visa-resource-name>)  [unwired: 1 in, 2 out]
            n1452 = Reciprocal(x="Flush rate (uL/m) P1") -> (1/x=w2045:dbl)
            n1453 = Number To Decimal String(number="Volume (uL) P1") -> (decimal integer string=w2053:string)  [unwired: 1 in]
            n1454 = Multiply(x="Volume (uL) P1", y=w2045) -> (x*y=w2044:dbl)
            n1455 = Concatenate Strings("tvolume  " ("string"), w2053, " u" ("string"), "\r") -> (w2051:string)
            n1456 = Multiply(x=w2044, y=60.0) -> (x*y=→"HP1 Flush Time (s)":dbl)
            n1457 = VISA Write(VISA resource name=w2062, write buffer=w2051) -> (VISA resource name out=w2050:refnum<visa-resource-name>)  [unwired: 1 in, 2 out]
            n1458 = Concatenate Strings("cvolume" ("string"), "\r") -> (w2049:string)
            n1459 = VISA Write(VISA resource name=w2050, write buffer=w2049) -> (VISA resource name out=w2060:refnum<visa-resource-name>)  [unwired: 1 in, 2 out]
            n1460 = Concatenate Strings("irun" ("string"), "\r") -> (w2058:string)
            n1461 = VISA Write(VISA resource name=w2060, write buffer=w2058) -> (VISA resource name out=w2048:refnum<visa-resource-name>)  [unwired: 1 in, 2 out]
          }
          frame #1 {
            "Flushing P1" <- TRUE ("Flushing P3")
          }
        }
      }
      event "Clear Volume": Value Change {
        n1462 = event-data() -> ()  [unwired: 7 out]
        n1463 = Number To Decimal String(number="Normal volume (mL)") -> (decimal integer string=w2073:string)  [unwired: 1 in]
        n1464 = Concatenate Strings("tvolume " ("string"), w2073, " u" ("string"), "\r") -> (w2070:string)
        n1465 = VISA Write(VISA resource name=w2076, write buffer=w2070) -> (VISA resource name out=w2069:refnum<visa-resource-name>)  [unwired: 1 in, 2 out]
        n1466 = local write "Clear Volume"(FALSE ("Clear Volume")) -> ()
        n1467 = Concatenate Strings("cvolume" ("string"), "\r") -> (w2078:string)
        n1468 = VISA Write(VISA resource name=w2069, write buffer=w2078) -> ()  [unwired: 1 in, 3 out]
      }
      event "Clear Volume P3": Value Change {
        n1469 = event-data() -> ()  [unwired: 7 out]
        n1470 = Concatenate Strings("cvolume" ("string"), "\r") -> (w2084:string)
        n1471 = VISA Write(VISA resource name=w2083, write buffer=w2084) -> ()  [unwired: 1 in, 3 out]
        n1472 = local write "Clear Volume P3"(FALSE ("Clear Volume P3")) -> ()
      }
      event "Clear Volume P1": Value Change {
        n1473 = event-data() -> ()  [unwired: 7 out]
        n1474 = Concatenate Strings("cvolume" ("string"), "\r") -> (w2089:string)
        n1475 = local write "Clear Volume P1"(FALSE ("Clear Volume P1")) -> ()
        n1476 = VISA Write(VISA resource name=w2088, write buffer=w2089) -> ()  [unwired: 1 in, 3 out]
      }
      event "Display On P3": Value Change {
        n1477 = event-data() -> ()  [unwired: 7 out]
        n1478 = Select(t="dim 100", s="Display On P3", f="dim 0") -> (s? t:f=w2095:string)
        n1479 = Concatenate Strings(w2095, "\r") -> (w2097:string)
        n1480 = VISA Write(VISA resource name=w2092, write buffer=w2097) -> ()  [unwired: 1 in, 3 out]
      }
      event "Display On P1": Value Change {
        n1481 = event-data() -> ()  [unwired: 7 out]
        n1482 = Select(t="dim 100", s="Display On P1", f="dim 0") -> (s? t:f=w2102:string)
        n1483 = Concatenate Strings(w2102, "\r") -> (w2104:string)
        n1484 = VISA Write(VISA resource name=w2099, write buffer=w2104) -> ()  [unwired: 1 in, 3 out]
      }
      event "Retract Pump 3": Value Change {
        n1485 = event-data() -> ()  [unwired: 7 out]
        n1486 = local write "Retract Pump 3"(FALSE ("Retract Pump 3")) -> ()
        n1487 = case shown="True" "Retract Pump 3" {
          tunnel: w2106 -> [_ w2109]
          frame False {
          }
          frame True {
            n1488 = Number To Decimal String(number="Retract Rate (mL/m)") -> (decimal integer string=w2127:string)  [unwired: 1 in]
            n1489 = Concatenate Strings("wrate  " ("string"), w2127, " u/m" ("string"), "\r") -> (w2129:string)
            n1490 = VISA Write(VISA resource name=w2109, write buffer=w2129) -> (VISA resource name out=w2120:refnum<visa-resource-name>)  [unwired: 1 in, 2 out]
            n1491 = Number To Decimal String(number="Retract Vol 3 (uL)") -> (decimal integer string=w2122:string)  [unwired: 1 in]
            n1492 = Concatenate Strings("tvolume  " ("string"), w2122, " u" ("string"), "\r") -> (w2119:string)
            n1493 = VISA Write(VISA resource name=w2120, write buffer=w2119) -> (VISA resource name out=w2115:refnum<visa-resource-name>)  [unwired: 1 in, 2 out]
            n1494 = Concatenate Strings("cvolume" ("string"), "\r") -> (w2116:string)
            n1495 = VISA Write(VISA resource name=w2115, write buffer=w2116) -> (VISA resource name out=w2110:refnum<visa-resource-name>)  [unwired: 1 in, 2 out]
            n1496 = Concatenate Strings("wrun" ("string"), "\r") -> (w2111:string)
            n1497 = VISA Write(VISA resource name=w2110, write buffer=w2111) -> ()  [unwired: 1 in, 3 out]
          }
        }
      }
      event "Retract Pump 1": Value Change {
        n1498 = event-data() -> ()  [unwired: 7 out]
        n1499 = local write "Retract Pump 1"(FALSE ("Retract Pump 1")) -> ()
        n1500 = case shown="True" "Retract Pump 1" {
          tunnel: w2131 -> [_ w2136]
          frame False {
          }
          frame True {
            n1501 = local read "Retract Rate (mL/m)"() -> (w2134:dbl)
            n1502 = Number To Decimal String(number=w2134) -> (decimal integer string=w2152:string)  [unwired: 1 in]
            n1503 = Concatenate Strings("wrate  " ("string"), w2152, " u/m" ("string"), "\r") -> (w2154:string)
            n1504 = VISA Write(VISA resource name=w2136, write buffer=w2154) -> (VISA resource name out=w2146:refnum<visa-resource-name>)  [unwired: 1 in, 2 out]
            n1505 = Number To Decimal String(number="Retract Vol 1 (uL)") -> (decimal integer string=w2148:string)  [unwired: 1 in]
            n1506 = Concatenate Strings("tvolume  " ("string"), w2148, " u" ("string"), "\r") -> (w2145:string)
            n1507 = VISA Write(VISA resource name=w2146, write buffer=w2145) -> (VISA resource name out=w2142:refnum<visa-resource-name>)  [unwired: 1 in, 2 out]
            n1508 = Concatenate Strings("cvolume" ("string"), "\r") -> (w2143:string)
            n1509 = VISA Write(VISA resource name=w2142, write buffer=w2143) -> (VISA resource name out=w2137:refnum<visa-resource-name>)  [unwired: 1 in, 2 out]
            n1510 = Concatenate Strings("wrun" ("string"), "\r") -> (w2138:string)
            n1511 = VISA Write(VISA resource name=w2137, write buffer=w2138) -> ()  [unwired: 1 in, 3 out]
          }
        }
      }
      event "Flip Green Filter": Value Change {
        n1512 = event-data() -> ()  [unwired: 7 out]
        n1513 = Not(x="Flip Green Filter") -> (.not. x?=w2156:bool)
        n1514 = local write "Flip Green Filter"(w2156) -> ()
        n1515 = flat-sequence {
          tunnel: w2164 -> [w2169]
          tunnel: w2163 -> [w2168]
          tunnel: [w2166] -> w2161
          tunnel: [w2165] -> w2160
          tunnel: [w2171] -> w2159
          tunnel: w2161 -> [w2171]
          tunnel: [w2170] -> w2158
          tunnel: w2160 -> [w2170]
          tunnel: w2159 -> [w2175]
          tunnel: w2158 -> [w2174]
          tunnel: [w2173] -> w2162
          frame #0 {
            n1516 = xnode "Read/Write Control"("FPGA VI Reference In"=w2169, "error in"=w2168, "Green Filter Flipper"=TRUE) -> ("FPGA VI Reference Out"=w2166:T19, "error out"=w2165:errorcluster)
          }
          frame #1 {
            n1517 = Wait (ms)(milliseconds to wait=u32 100) -> ()  [unwired: 1 out]
          }
          frame #2 {
            n1518 = xnode "Read/Write Control"("FPGA VI Reference In"=w2175, "error in"=w2174, "Green Filter Flipper"=FALSE) -> ("error out"=w2173:errorcluster)  [unwired: 1 out]
          }
        }
      }
      event "Pump 1 contents", "Pump 3 contents": Value Change {
        n1519 = event-data() -> ()  [unwired: 7 out]
        n1520 = local read "Pump 1 contents"() -> (→"Pump 1 cont disp":string)
        n1521 = local read "Pump 3 contents"() -> (→"Pump 3 cont disp":string)
      }
      event "Reset Trap Pos. FB": Value Change {
        n1522 = event-data() -> ()  [unwired: 7 out]
        n1523 = xnode "Read/Write Control"("FPGA VI Reference In"=w2181, "error in"=w2180, "Trap Pos. FB Reset"="Reset Trap Pos. FB") -> ()  [unwired: 2 out]
      }
      event "Rem fb disp offset": Value Change {
        n1524 = event-data() -> ()  [unwired: 7 out]
        n1525 = local write "Rem fb disp offset"(FALSE ("Rem fb disp offset")) -> ()
        n1526 = local read "Mean T1 Position (nm)"() -> (w2183:dbl)
        n1527 = local read "FB Trap Pos Offset"() -> (w2184:dbl)
        n1528 = Subtract(x=w2184, y=w2183) -> (x-y=w2182:dbl)
        n1529 = local write "FB Trap Pos Offset"(w2182) -> ()
      }
      event "Threshold (nm)": Value Change {
        n1530 = event-data() -> ()  [unwired: 7 out]
        n1531 = flat-sequence {
          tunnel: w2188 -> [w2196]
          tunnel: w2187 -> [w2195]
          tunnel: [w2189] -> w2186
          tunnel: w2186 -> [w2202]
          frame #0 {
            n1532 = xnode "Read/Write Control"("FPGA VI Reference In"=w2196, "error in"=w2195) -> ("FPGA VI Reference Out"=w2192:T19, "error out"=w2191:errorcluster, "FPGA TTrig Thresh"=w2193:i64)
            n1533 = local read "Threshold stored (nm)"() -> (w2201:dbl)
            n1534 = local read "Threshold (nm)"() -> (w2189:dbl)
            n1535 = local read "AOM X Cal (nm/MHz)"() -> (w2199:dbl)
            n1536 = Subtract(x=w2189, y=w2201) -> (x-y=w2200:dbl)
            n1537 = Divide(x=w2200, y=w2199) -> (x/y=w2197:dbl)
            n1538 = call "IR AOM freq to word.vi"("Frequency In (MHz)"=w2197) -> ("Frequency Word Out (double)"=w2198:dbl)
            n1539 = To Quad Integer(1:w2198) -> (0:w2194:i64)
            n1540 = Add(x=w2193, y=w2194) -> (x+y=w2190:i64)
            n1541 = xnode "Read/Write Control"("FPGA VI Reference In"=w2192, "error in"=w2191, "FPGA TTrig Thresh"=w2190) -> ()  [unwired: 2 out]
          }
          frame #1 {
            "Threshold stored (nm)" <- w2202
          }
        }
      }
      event "FB Trig Integrate": Value Change {
        n1542 = event-data() -> ()  [unwired: 7 out]
        n1543 = local read "FB Trig Integrate"() -> (w2204:u32)
        n1544 = xnode "Read/Write Control"("FPGA VI Reference In"=w2206, "error in"=w2205, "FB Trig Integrate"=w2204) -> ("error out"=w2203:errorcluster)  [unwired: 1 out]
      }
      event "11": Value Change {
        n1545 = event-data() -> ()  [unwired: 7 out]
        n1546 = local read "11"() -> (w2207:bool)
        n1547 = case shown="True" w2207 {
          frame False {
          }
          frame True {
            n1548 = local read "Messages"() -> (w2209:string)
            n1549 = call "Update messages.vi"("Message to add"="You kicked it up to 11!", "Old message string"=w2209) -> ("New message string"=w2210:string)
            n1550 = call <vilib>:"Beep.vi"() -> ()  [unwired: 12 in]
            n1551 = local write "Messages"(w2210) -> ()
          }
        }
      }
      event "Trap Pos. FB ON": Value Change {
        n1552 = event-data() -> ()  [unwired: 7 out]
        n1553 = xnode "Read/Write Control"("FPGA VI Reference In"=w2213, "error in"=w2212, "Force feedback"="Trap Pos. FB ON") -> ()  [unwired: 2 out]
      }
      event "Remove Action Offset": Value Change {
        n1554 = event-data() -> ()  [unwired: 7 out]
        n1555 = local write "Remove Action Offset"(FALSE ("Remove Action Offset")) -> ()
        n1556 = local read "Trap Pos. FB Mult Factor"() -> (w2218:i64)
        n1557 = local read "Trap Pos FB Action"() -> (w2216:i64)
        n1558 = local read "Trap Pos. FB Offset Factor"() -> (w2214:i64)
        n1559 = Multiply(x=w2218, y=w2216) -> (x*y=w2217:i64)
